vi "String mit Leerzeichen auffuellen.vi"(8 "2 Dimension":string[][](array[string]), 10 "1 Dimension":string[](array[string]), 11 "gewünschte Stringgröße":i32=11) -> (0 "2 Dimension":string[][](array[string]), 2 "1 Dimension":string[](array[string]))   [LabVIEW 2020, in "Linearisierung v2.lvlib" / "Linearity verification 1065-307.lvlib"]
uses:
  Linearity verification 1065-307.lvlib
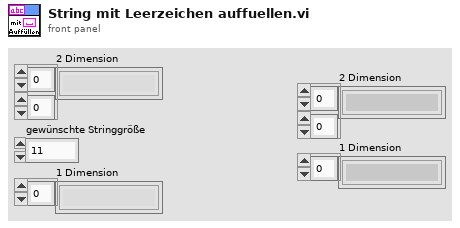
[diagram p1: front panel]
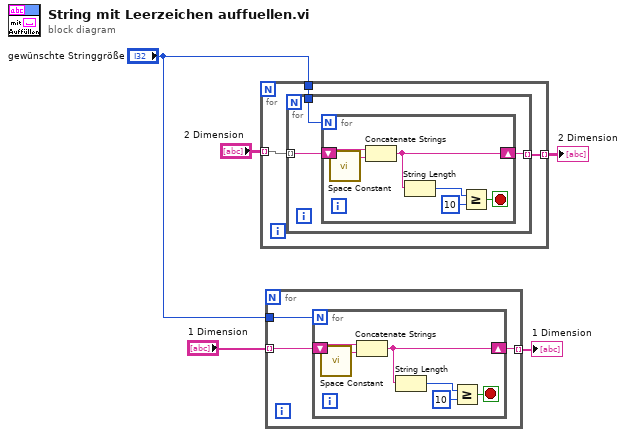
[diagram p0: block diagram]
diagram:
  n1 = for {
    tunnel: "2 Dimension" -> [w8] mode=indexing
    tunnel: [w7] -> w4 mode=indexing
    tunnel: "gewünschte Stringgröße" -> [w6]
    n2 = for {
      tunnel: w8 -> [w11] mode=indexing
      tunnel: [w10] -> w7 mode=indexing
      tunnel: w6 -> [w9]
      n3 = for {
        N: w9 -> [_]
        shift-right: [w15] -> w10
        shift-left: w11 -> [w17]
        stop <- w12 stop-if-true
        n4 = call <vilib>:"Space Constant.vi"() -> ("String"=w16:string)
        n5 = Concatenate Strings(w17, w16) -> (w15:string)
        n6 = String Length(string=w15) -> (length=w14:i32)
        n7 = Greater Or Equal?(x=w14, y=10) -> (x >= y?=w12:bool)
      }
    }
  }
  "2 Dimension" <- w4
  n8 = for {
    tunnel: "1 Dimension" -> [w20] mode=indexing
    tunnel: [w19] -> w2 mode=indexing
    tunnel: "gewünschte Stringgröße" -> [w18]
    n9 = for {
      N: w18 -> [_]
      shift-right: [w24] -> w19
      shift-left: w20 -> [w26]
      stop <- w21 stop-if-true
      n10 = call <vilib>:"Space Constant.vi"() -> ("String"=w25:string)
      n11 = Concatenate Strings(w26, w25) -> (w24:string)
      n12 = String Length(string=w24) -> (length=w23:i32)
      n13 = Greater Or Equal?(x=w23, y=10) -> (x >= y?=w21:bool)
    }
  }
  "1 Dimension" <- w2
